vi "Create Table.vi"(7 "Cluster In":variant, 8 "error in (no error)":errorcluster, 10 "Table Name":string, 11 "PostgreSQL in":refnum<class "PostgreSQL.lvclass">) -> (0 "error out":errorcluster, 1 "Column Names":string[](array[string]), 2 "Table Name out":string, 3 "PostgreSQL out":refnum<class "PostgreSQL.lvclass">)   [LabVIEW 2018, in "Database.lvlib" / "PostgreSQL.lvclass"]
uses:
  PostgreSQL.lvclass
  DatabaseBaseClass/DatabaseBaseClass.lvclass
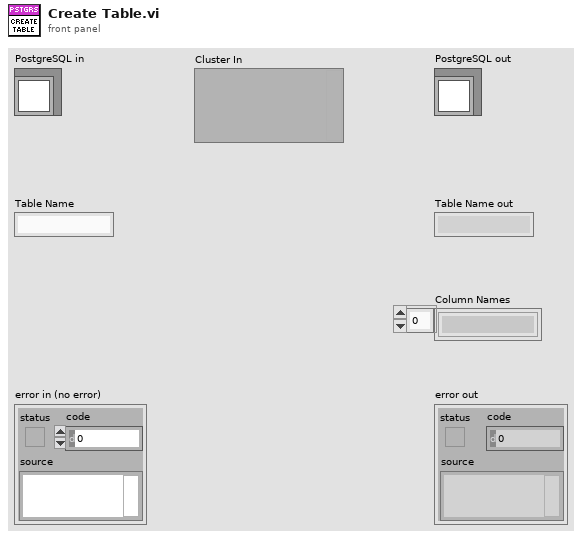
[diagram p1: front panel]
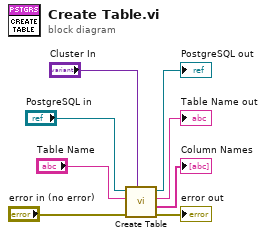
[diagram p0: block diagram]
diagram:
  n1 = call-parent "Create Table.vi"("Cluster In"="Cluster In", "error in (no error)"="error in (no error)", "Table Name"="Table Name", "DatabaseBaseClass In"="PostgreSQL in") -> ("error out"=→"error out":errorcluster, "Column Names"=→"Column Names":string[], "Table Name out"=→"Table Name out":string, "DatabaseBaseClass out"=→"PostgreSQL out":refnum<class "PostgreSQL.lvclass">)  [unwired: 4 in]
